vi "Robot Global Data.vi"() -> ()   [LabVIEW 2013]
doc: "This global VI can contain as many global variables as you need. Place a control on the panel, give it a good name. To read or write to it from a VI, drag the icon to the diagram of that VI. You can also drag from the project. Click on the node to change which global you access. You shouldn't have multiple locations writing to a global or it will cause a race-condition."
uses:
  <vilib>/Rock Robotics/WPI/Camera/WPI_CameraImageSize.ctl
  <vilib>/Rock Robotics/WPI/DriverStation/WPI_DriverStationRobotMode2.ctl
  User Commands typedef.ctl
  Arm control typedef.ctl
  Arm Postions Enum Typedef.ctl
  Shooter Commands Typedef.ctl
  Drive Commands Typedef.ctl
  Robot Info Typedef.ctl
  Arm Info Typedef.ctl
  Shooter Info Typedef.ctl
  Shooter State Enum.ctl
  Arm State Enum Typedef.ctl
panel:
  in  "Arm State":T1
  in  "Shooter State":T2=enum."Fired"
  in  "Robot Info":T3
  in  "User Commands":T6
  in  "Robot Mode":T11
  in  "LED toggle rate (ms)":u32=20
  in  "image size":T12=enum."320x240"
  in  "Enable Vision":bool
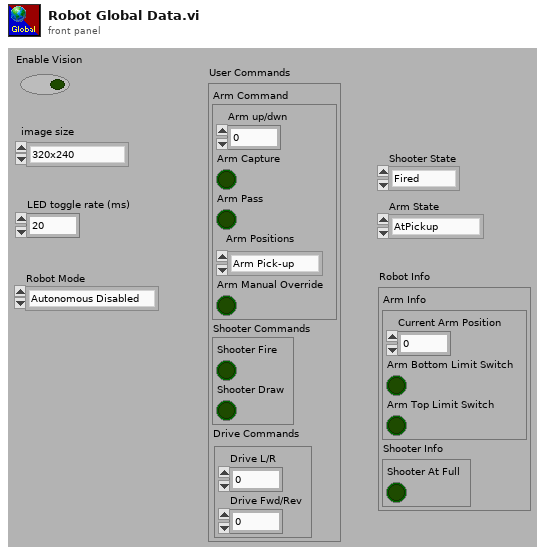
[diagram p1: front panel]
types:
  T1 = typedef "Arm State Enum Typedef.ctl" = enum16{"AtPickup", "MovingDownToPickup", "MovingUpToShoot", "AtShoot", "MovingDownToShoot", "MovingUpToTruss", "AtTruss"}
  T2 = typedef "Shooter State Enum.ctl" = enum16{"Ready", "Fired", "DrawingToReady"}
  T3 = typedef "Robot Info Typedef.ctl" = cluster{"Arm Info":T4, "Shooter Info":T5}
  T4 = typedef "Arm Info Typedef.ctl" = cluster{"Current Arm Position":dbl, "Arm Bottom Limit Switch":bool, "Arm Top Limit Switch":bool}
  T5 = typedef "Shooter Info Typedef.ctl" = cluster{"Shooter At Full":bool}
  T6 = typedef "User Commands typedef.ctl" = cluster{"Arm Command":T7, "Shooter Commands":T9, "Drive Commands":T10}
  T7 = typedef "Arm control typedef.ctl" = cluster{"Arm up/dwn":dbl, "Arm Capture":bool, "Arm Pass":bool, "Arm Positions":T8, "Arm Manual Override":bool}
  T8 = typedef "Arm Postions Enum Typedef.ctl" = enum16{"Arm Pick-up", "Idle", "Arm Shoot", "Arm Truss", "Manual"}
  T9 = typedef "Shooter Commands Typedef.ctl" = cluster{"Shooter Fire":bool, "Shooter Draw":bool}
  T10 = typedef "Drive Commands Typedef.ctl" = cluster{"Drive L/R":dbl, "Drive Fwd/Rev":dbl}
  T11 = typedef "WPI_DriverStationRobotMode2.ctl" = enum16{"Autonomous Disabled", "Autonomous Enabled", "Teleop Disabled", "Teleop Enabled", "Timeout", "Finish", "Test Disabled", "Test Enabled"}
  T12 = typedef "WPI_CameraImageSize.ctl" = enum16{"640x480", "320x240", "160x120"}
diagram:
